vi "PWM Config.vi"(8 "error in (no error)":errorcluster, 11 "FileConfig in":refnum<class "FileConfig.lvclass">) -> (0 "error out":errorcluster, 1 "IDs found?":bool, 2 "PWM Data":T1, 3 "FileConfig out":refnum<class "FileConfig.lvclass">, 5 "File Found?":bool)   [LabVIEW 2019, in "Config.lvlib" / "FileConfig.lvclass"]
doc: "Use this VI to retrieve the PWM channels that will be used in the robot."
uses:
  FileConfig.lvclass
  Config/Controls/PWM Data.ctl
  <vilib>/Rock Robotics/SystemInterfaces/DIO/FPGA_DIOPWMChannel.ctl
  FileConfig.lvclass/FileConfig.ctl
  Config.lvclass
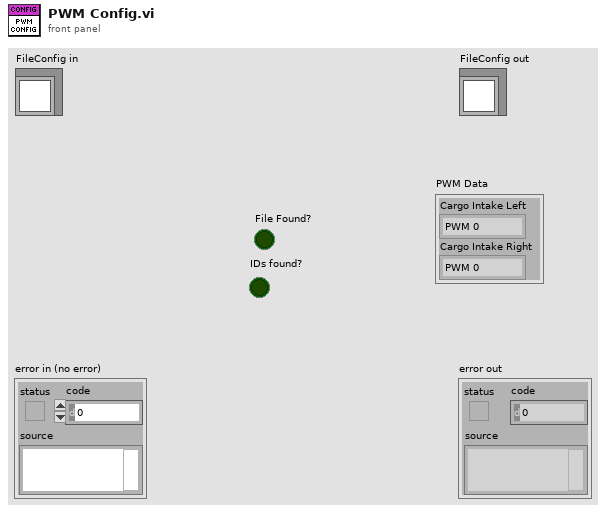
[diagram p1: front panel]
types:
  T1 = typedef "Config.lvlib/Config.lvclass/PWM Data.ctl" = cluster{"Cargo Intake Left":T2, "Cargo Intake Right":T2}
  T2 = typedef "FPGA_DIOPWMChannel.ctl" = enum8{"PWM 0", "PWM 1", "PWM 2", "PWM 3", "PWM 4", "PWM 5", "PWM 6", "PWM 7", "PWM 8", "PWM 9", "PWM MXP 0", "PWM MXP 1", "PWM MXP 2", "PWM MXP 3", "PWM MXP 4", "PWM MXP 5", "PWM MXP 6", "PWM MXP 7", "PWM MXP 8", "PWM MXP 9", "Invalid"}
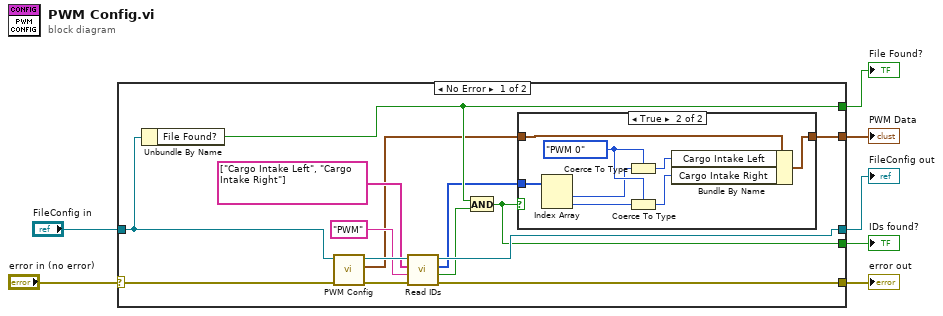
[diagram p0: block diagram]
diagram:
  n1 = case shown="No Error" "error in (no error)" {
    selector: "error in (no error)" -> [w20 w32]
    tunnel: [w18 w32] -> w7
    tunnel: [w8 _] -> w6
    tunnel: [w9 _] -> w5
    tunnel: [w16 w31] -> w4
    tunnel: [w13 _] -> w3
    tunnel: "FileConfig in" -> [w19 w31]
    frame No Error {
      n2 = Unbundle By Name(w19) -> ("File Found?"=w13:bool)
      n3 = call-parent "PWM Config.vi"("error in (no error)"=w20, "Config in"=w19) -> ("error out"=w21:errorcluster, "PWM Data"=w10:T1, "Config out"=w17:refnum<class "FileConfig.lvclass">)  [unwired: 5 in, 2 out]
      n4 = call "Read IDs.vi"("error in (no error)"=w21, "section"="PWM", "keys"=string[] ["Cargo Intake Left", "Cargo Intake Right"], "FileConfig in"=w17) -> ("error out"=w18:errorcluster, "Found?"=w12:bool, "Found IDs"=w11:u8[], "FileConfig out"=w16:refnum<class "FileConfig.lvclass">)  [unwired: 4 in]
      n5 = And(x=w13, y=w12) -> (x .and. y?=w8:bool)
      n6 = case shown="True" w8 {
        tunnel: w11 -> [_ w28]
        tunnel: w10 -> [w22 w30]
        tunnel: [w22 w29] -> w9
        frame False {
        }
        frame True {
          w27 = FPGA_DIOPWMChannel."PWM 0" ("Cargo Intake Right")
          n7 = Index Array(array=w28) -> (element #1=w25:u8, element #2=w26:u8)  [unwired: 2 in]
          n8 = Coerce To Type(0:w25, 1:w27) -> (2:w24:T2)
          n9 = Coerce To Type(0:w26, 1:w27) -> (2:w23:T2)
          n10 = Bundle By Name(cluster=w30, "Cargo Intake Left"=w24, "Cargo Intake Right"=w23) -> (w29:T1)
        }
      }
    }
    frame Error {
    }
  }
  "error out" <- w7
  "FileConfig out" <- w4
  "File Found?" <- w3
  "IDs found?" <- w6
  "PWM Data" <- w5
